vi "GlobalMulticast.vi"() -> ()   [LabVIEW 2017, in "LV_Unicorn.lvlib"]
uses:
  LV_Unicorn.lvlib
  Control/AnswerUDP.ctl
panel:
  in  "net address":u32
  in  "modbustype, version":u32=4294967295 format="%08x"
  in  "VersionControl":bool=TRUE
  out "tblT":string[][](table) caption="Найденные устройства."
  out "devT":T1[](array[typedef])
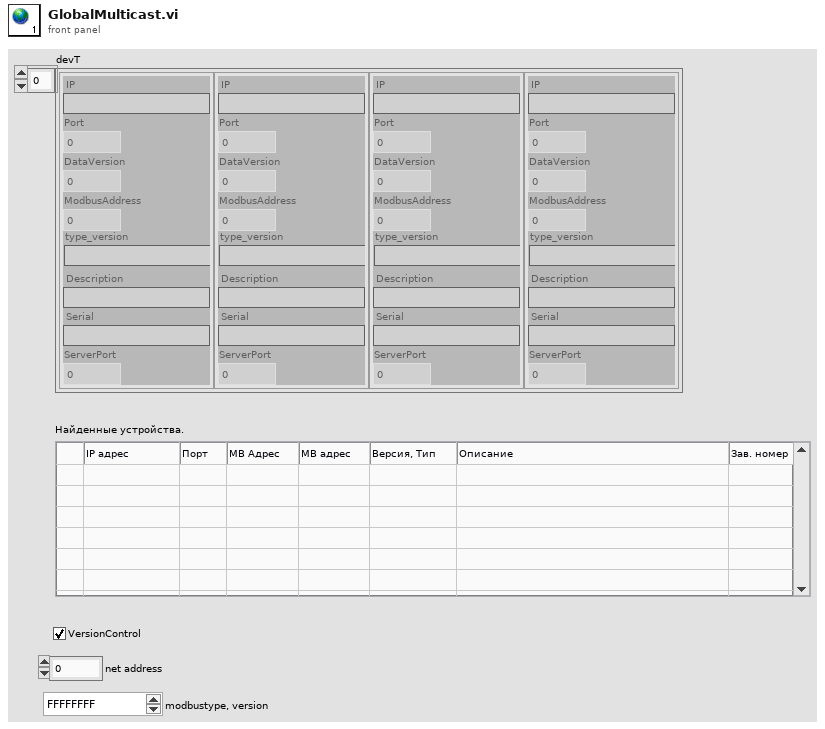
[diagram p1: front panel]
types:
  T1 = typedef "LV_Unicorn.lvlib/AnswerUDP.ctl" = cluster{"IP":string, "Port":u16, "DataVersion":u16, "ModbusAddress":i32, "type_version":string, "Description":string, "Serial":string, "ServerPort":u16}
diagram:
